vi "Empty Panel 2.vi"   [LabVIEW 2014]
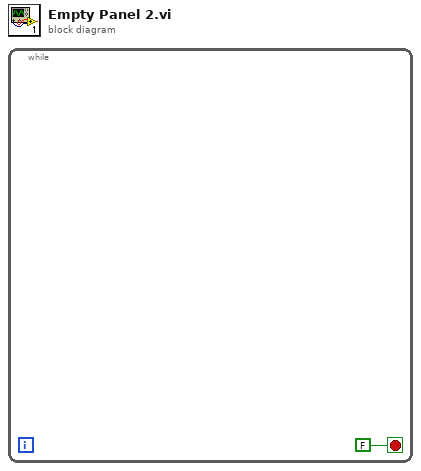
[diagram p0: block diagram]
diagram:
  n1 = while {
    stop <- FALSE stop-if-true
  }
